vi "Position_FBL.vi"() -> (1 "Z":dbl, 2 "Y":dbl, 3 "X":dbl)   [LabVIEW 2019]
uses:
  <userlib>/HapticSTM/HapticSTM.lvlib
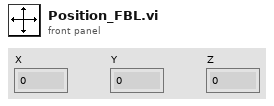
[diagram p1: front panel]
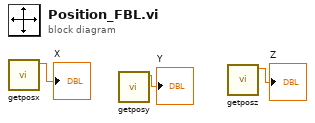
[diagram p0: block diagram]
diagram:
  n1 = call <userlib>:"getposx.vi"() -> ("function return"=→"X":dbl)  [unwired: 11 in]
  n2 = call <userlib>:"getposy.vi"() -> ("function return"=→"Y":dbl)  [unwired: 11 in]
  n3 = call <userlib>:"getposz.vi"() -> ("function return"=→"Z":dbl)  [unwired: 11 in]
